vi "ARINC 429 - Add Single TimeStamp Channel.vi"(8 "error in (no error)":errorcluster, 11 "Node Ptr":u64 format="%.0x") -> (0 "error out":errorcluster)   [LabVIEW 2015, in "AIT 429 System Explorer.lvlib"]
doc: "Add timestamp channel for the selected label"
uses:
  AIT 429 System Explorer.lvlib
  Shared/Controls and Global/Global.vi
  <vilib>/NI Veristand/Custom Device Tools/Custom Device Utility Library/NI VeriStand - Search for Item by GUID.vi
  <vilib>/NI VeriStand/Custom Device API/Custom Device API.lvlib
  <vilib>/NI VeriStand/Custom Device Tools/Custom Device Utility Library/Custom Device Utility Library.lvlib
  Shared/ARINC 429 Shared.lvlib
panel:
  in  "Tag":string
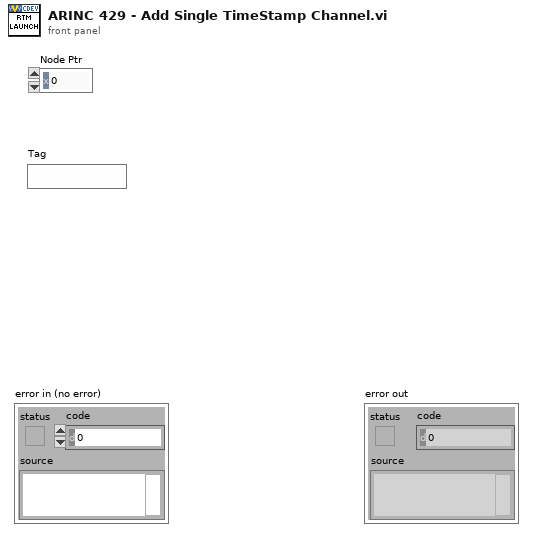
[diagram p1: front panel]
types:
  T1 = typedef "Custom Device API.lvlib/Custom Device Item Ref.ctl" = u64
  T2 = typedef "Custom Device API.lvlib/Custom Device Item Info.ctl" = cluster{"Name":string, "Is Channel":bool, "GUID":string, "Is Waveform":bool}
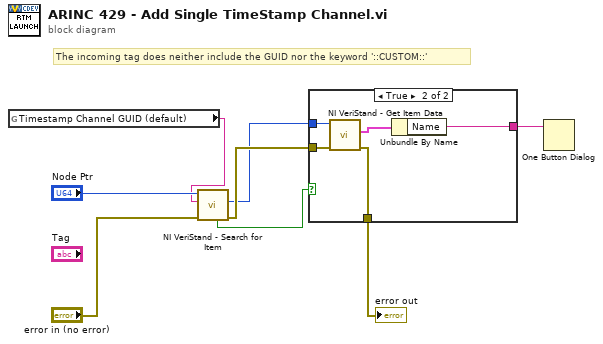
[diagram p0: block diagram]
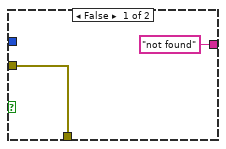
[diagram p2: hidden frame]
diagram:
  # "The incoming tag does neither include the GUID nor the keyword '::CUSTOM::'"
  n1 = global read "Global.vi" "Timestamp Channel GUID (default)"() -> (w7:string)
  n2 = call-poly <vilib>:"NI VeriStand - Search for Item.vi"("error in"="error in (no error)", "Item GUID"=w7, "Section Ref in"="Node Ptr") -> ("error out"=w5:errorcluster, "Item Ref"=w3:T1, "Found"=w2:bool)  [unwired: 5 in, 1 out]
  n3 = case shown="True" w2 {
    tunnel: w5 -> [w9 w15]
    tunnel: [w9 w14] -> w4
    tunnel: w3 -> [_ w13]
    tunnel: ["not found" ("Name") w11] -> w1
    frame False {
    }
    frame True {
      n4 = call <vilib>:"NI VeriStand - Get Item Data.vi"("error in (no error)"=w15, "Item Ref in"=w13) -> ("error out"=w14:errorcluster, "Item Info"=w12:T2)  [unwired: 6 in, 2 out]
      n5 = Unbundle By Name(w12) -> ("Name"=w11:string)
    }
  }
  "error out" <- w4
  n6 = One Button Dialog(message=w1) -> ()  [unwired: 1 in, 1 out]
